vi "generatePinnedRobots.vi"(8 "error in (no error)":errorcluster, 9 "Defensive ids":dbl[](array[numeric]), 10 "Offensive ids":dbl[](array[numeric]), 11 "Game in":refnum<class "Game.lvclass">) -> (0 "error out":errorcluster, 3 "Game out":refnum<class "Game.lvclass">)   [LabVIEW 2018, in "Game.lvclass"]
uses:
  Game.lvclass
  Utilities_class/Utilities.lvclass
  Ally_class/Ally.lvclass
  C:/Users/nicolas.oliveira/roboime/SSL_AI/Team_class/Team.lvclass
  Robot_class/Robot.lvclass
  Game.lvclass/Game.ctl
  Team_class/Team.lvclass/Team.ctl
  Robot_class/Robot.lvclass/Robot.ctl
  Robot_class/Read id.vi
  Read AllyRef.vi
  Team_class/Read RobotRef.vi
  Team_class/Write RobotRef.vi
  Write Pinned Deffensive.vi
  Write Pinned Offensive.vi
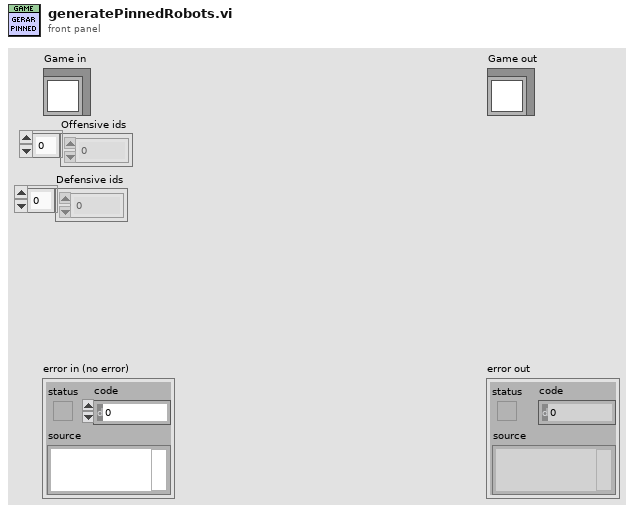
[diagram p1: front panel]
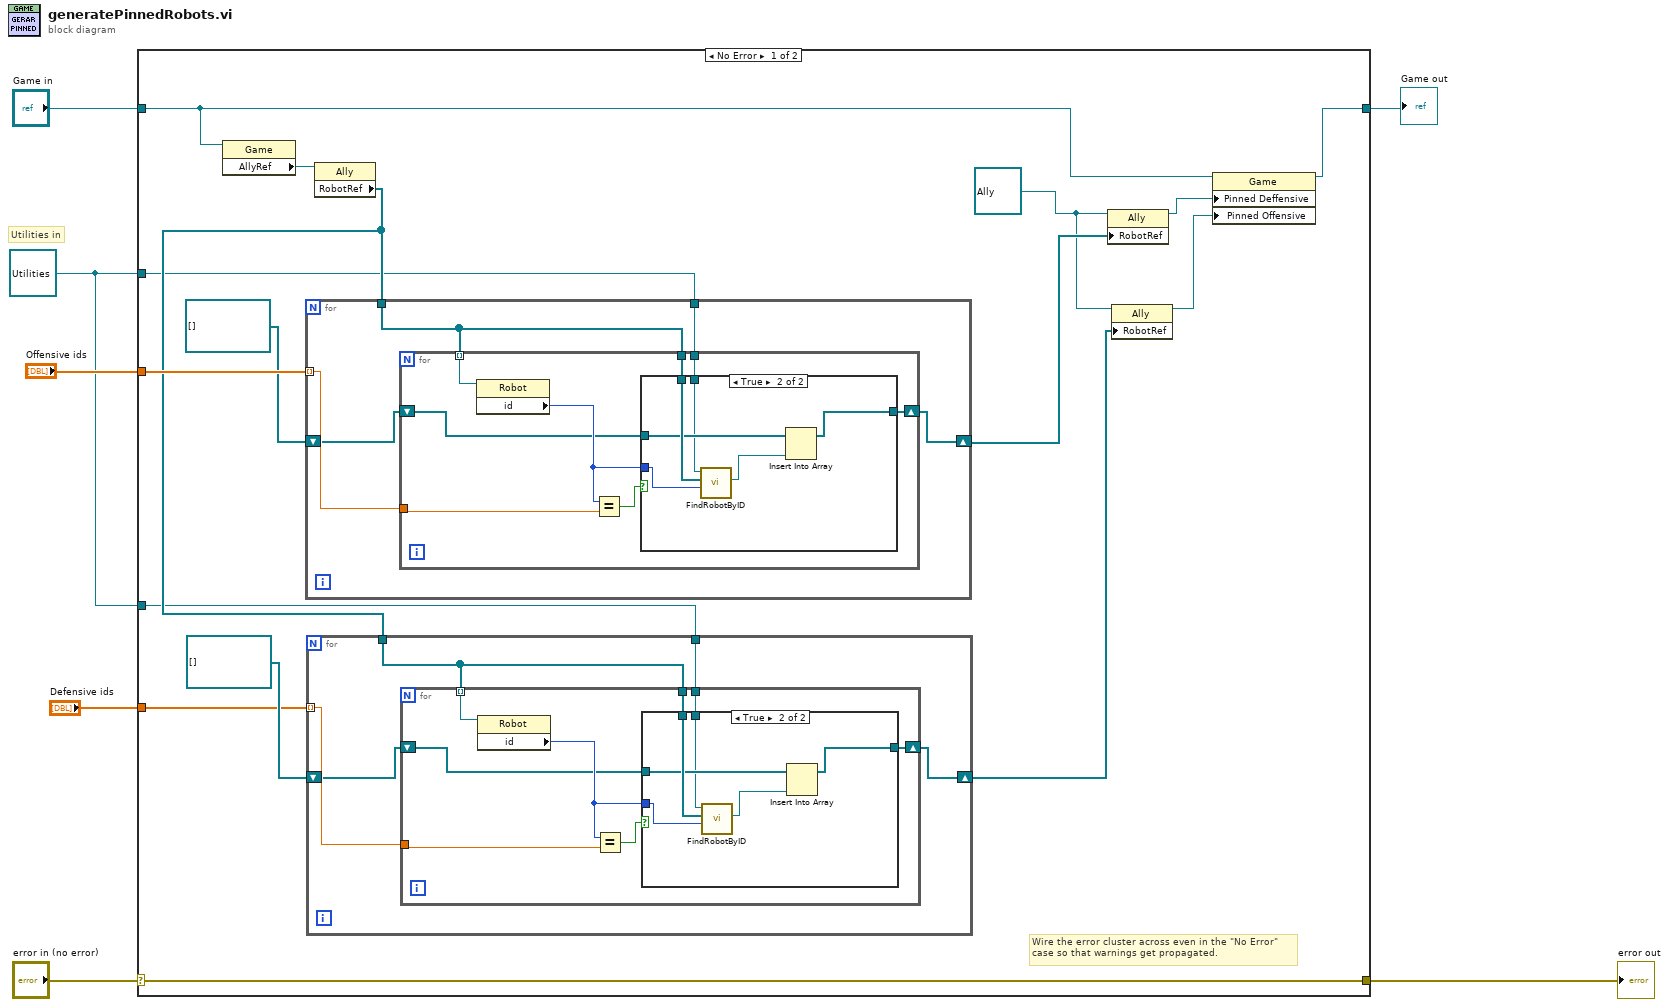
[diagram p0: block diagram]
diagram:
  w1 = refnum<class "Utilities.lvclass"> refnum ("Utilities in")
  # "Utilities in"
  n1 = case shown="No Error" "error in (no error)" {
    selector: "error in (no error)" -> [w23 w65]
    tunnel: [w23 w65] -> w6
    tunnel: [w12 w64] -> w4
    tunnel: "Game in" -> [w20 w64]
    tunnel: "Offensive ids" -> [w21 _]
    tunnel: "Defensive ids" -> [w14 _]
    tunnel: w1 -> [w10 _]
    tunnel: w1 -> [w8 _]
    frame No Error {
      w9 = refnum<class "Ally.lvclass"> refnum ("Pinned Deffensive")
      # "Wire the error cluster across even in the \"No Error\"\ncase so that warnings get propagated."
      n2 = property class="Game"(reference=w20) -> ("AllyRef"=w19:refnum<class "Ally.lvclass">)  [unwired: 1 in, 2 out]
      n3 = property class="Ally"(reference=w19) -> ("RobotRef"=w13:refnum<class "Robot.lvclass">[])  [unwired: 1 in, 2 out]
      n4 = for {
        tunnel: w21 -> [w48] mode=indexing
        tunnel: w13 -> [w47]
        shift-right: [w45] -> w17
        shift-left: refnum<class "Robot.lvclass">[] [] -> [w46]
        tunnel: w10 -> [w44]
        n5 = for {
          tunnel: w47 -> [w54] mode=indexing
          tunnel: w48 -> [w56]
          tunnel: w47 -> [w53]
          shift-right: [w51] -> w45
          shift-left: w46 -> [w50]
          tunnel: w44 -> [w49]
          n6 = property class="Robot"(reference=w54) -> ("id"=w52:i32)  [unwired: 1 in, 2 out]
          n7 = Equal?(x=w52, y=w56) -> (x = y?=w55:bool)
          n8 = case shown="True" w55 {
            tunnel: w53 -> [_ w63]
            tunnel: w52 -> [_ w62]
            tunnel: [w57 w60] -> w51
            tunnel: w50 -> [w57 w59]
            tunnel: w49 -> [_ w58]
            frame False {
            }
            frame True {
              n9 = call-dynamic "FindRobotByID.vi"("id"=w62, "RobotRef"=w63, "Utilities in"=w58) -> ("Robot"=w61:refnum<class "Robot.lvclass">)  [unwired: 5 in, 3 out]
              n10 = Insert Into Array(array=w59, new element=w61) -> (w60:refnum<class "Robot.lvclass">[])  [unwired: 1 in]
            }
          }
        }
      }
      n11 = for {
        tunnel: w14 -> [w28] mode=indexing
        tunnel: w13 -> [w27]
        shift-right: [w25] -> w11
        shift-left: refnum<class "Robot.lvclass">[] [] -> [w26]
        tunnel: w8 -> [w24]
        n12 = for {
          tunnel: w27 -> [w34] mode=indexing
          tunnel: w28 -> [w36]
          tunnel: w27 -> [w33]
          shift-right: [w31] -> w25
          shift-left: w26 -> [w30]
          tunnel: w24 -> [w29]
          n13 = property class="Robot"(reference=w34) -> ("id"=w32:i32)  [unwired: 1 in, 2 out]
          n14 = Equal?(x=w32, y=w36) -> (x = y?=w35:bool)
          n15 = case shown="True" w35 {
            tunnel: w33 -> [_ w43]
            tunnel: w32 -> [_ w42]
            tunnel: [w37 w40] -> w31
            tunnel: w30 -> [w37 w39]
            tunnel: w29 -> [_ w38]
            frame False {
            }
            frame True {
              n16 = call-dynamic "FindRobotByID.vi"("id"=w42, "RobotRef"=w43, "Utilities in"=w38) -> ("Robot"=w41:refnum<class "Robot.lvclass">)  [unwired: 5 in, 3 out]
              n17 = Insert Into Array(array=w39, new element=w41) -> (w40:refnum<class "Robot.lvclass">[])  [unwired: 1 in]
            }
          }
        }
      }
      n18 = property class="Ally"(reference=w9, "RobotRef"=w17) -> (reference out=w22:refnum<class "Ally.lvclass">)  [unwired: 1 in, 1 out]
      n19 = property class="Ally"(reference=w9, "RobotRef"=w11) -> (reference out=w16:refnum<class "Ally.lvclass">)  [unwired: 1 in, 1 out]
      n20 = property class="Game"(reference=w20, "Pinned Deffensive"=w22, "Pinned Offensive"=w16) -> (reference out=w12:refnum<class "Game.lvclass">)  [unwired: 1 in, 1 out]
    }
    frame Error {
    }
  }
  "error out" <- w6
  "Game out" <- w4
